vi "create_file_name (SubVI).vi"(0 "Use electrode config?":bool, 1 "Step Picomotors?":bool, 4 "picomotor index":i32, 6 "file_idx":i32, 8 "num files":i32, 9 "base name":string, 10 "Path":path, 11 "process_list":T2) -> (2 "filename_cluster":T1)   [LabVIEW 2018]
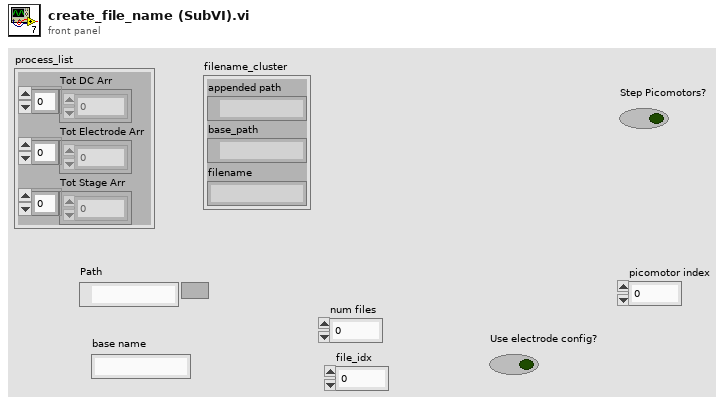
[diagram p1: front panel]
types:
  T1 = cluster{"appended path":path, "base_path":path, "filename":string}
  T2 = cluster{"Tot DC Arr":dbl[], "Tot Electrode Arr":dbl[], "Tot Stage Arr":dbl[]}
  T3 = cluster{"appended path":path, "path out":path, string}
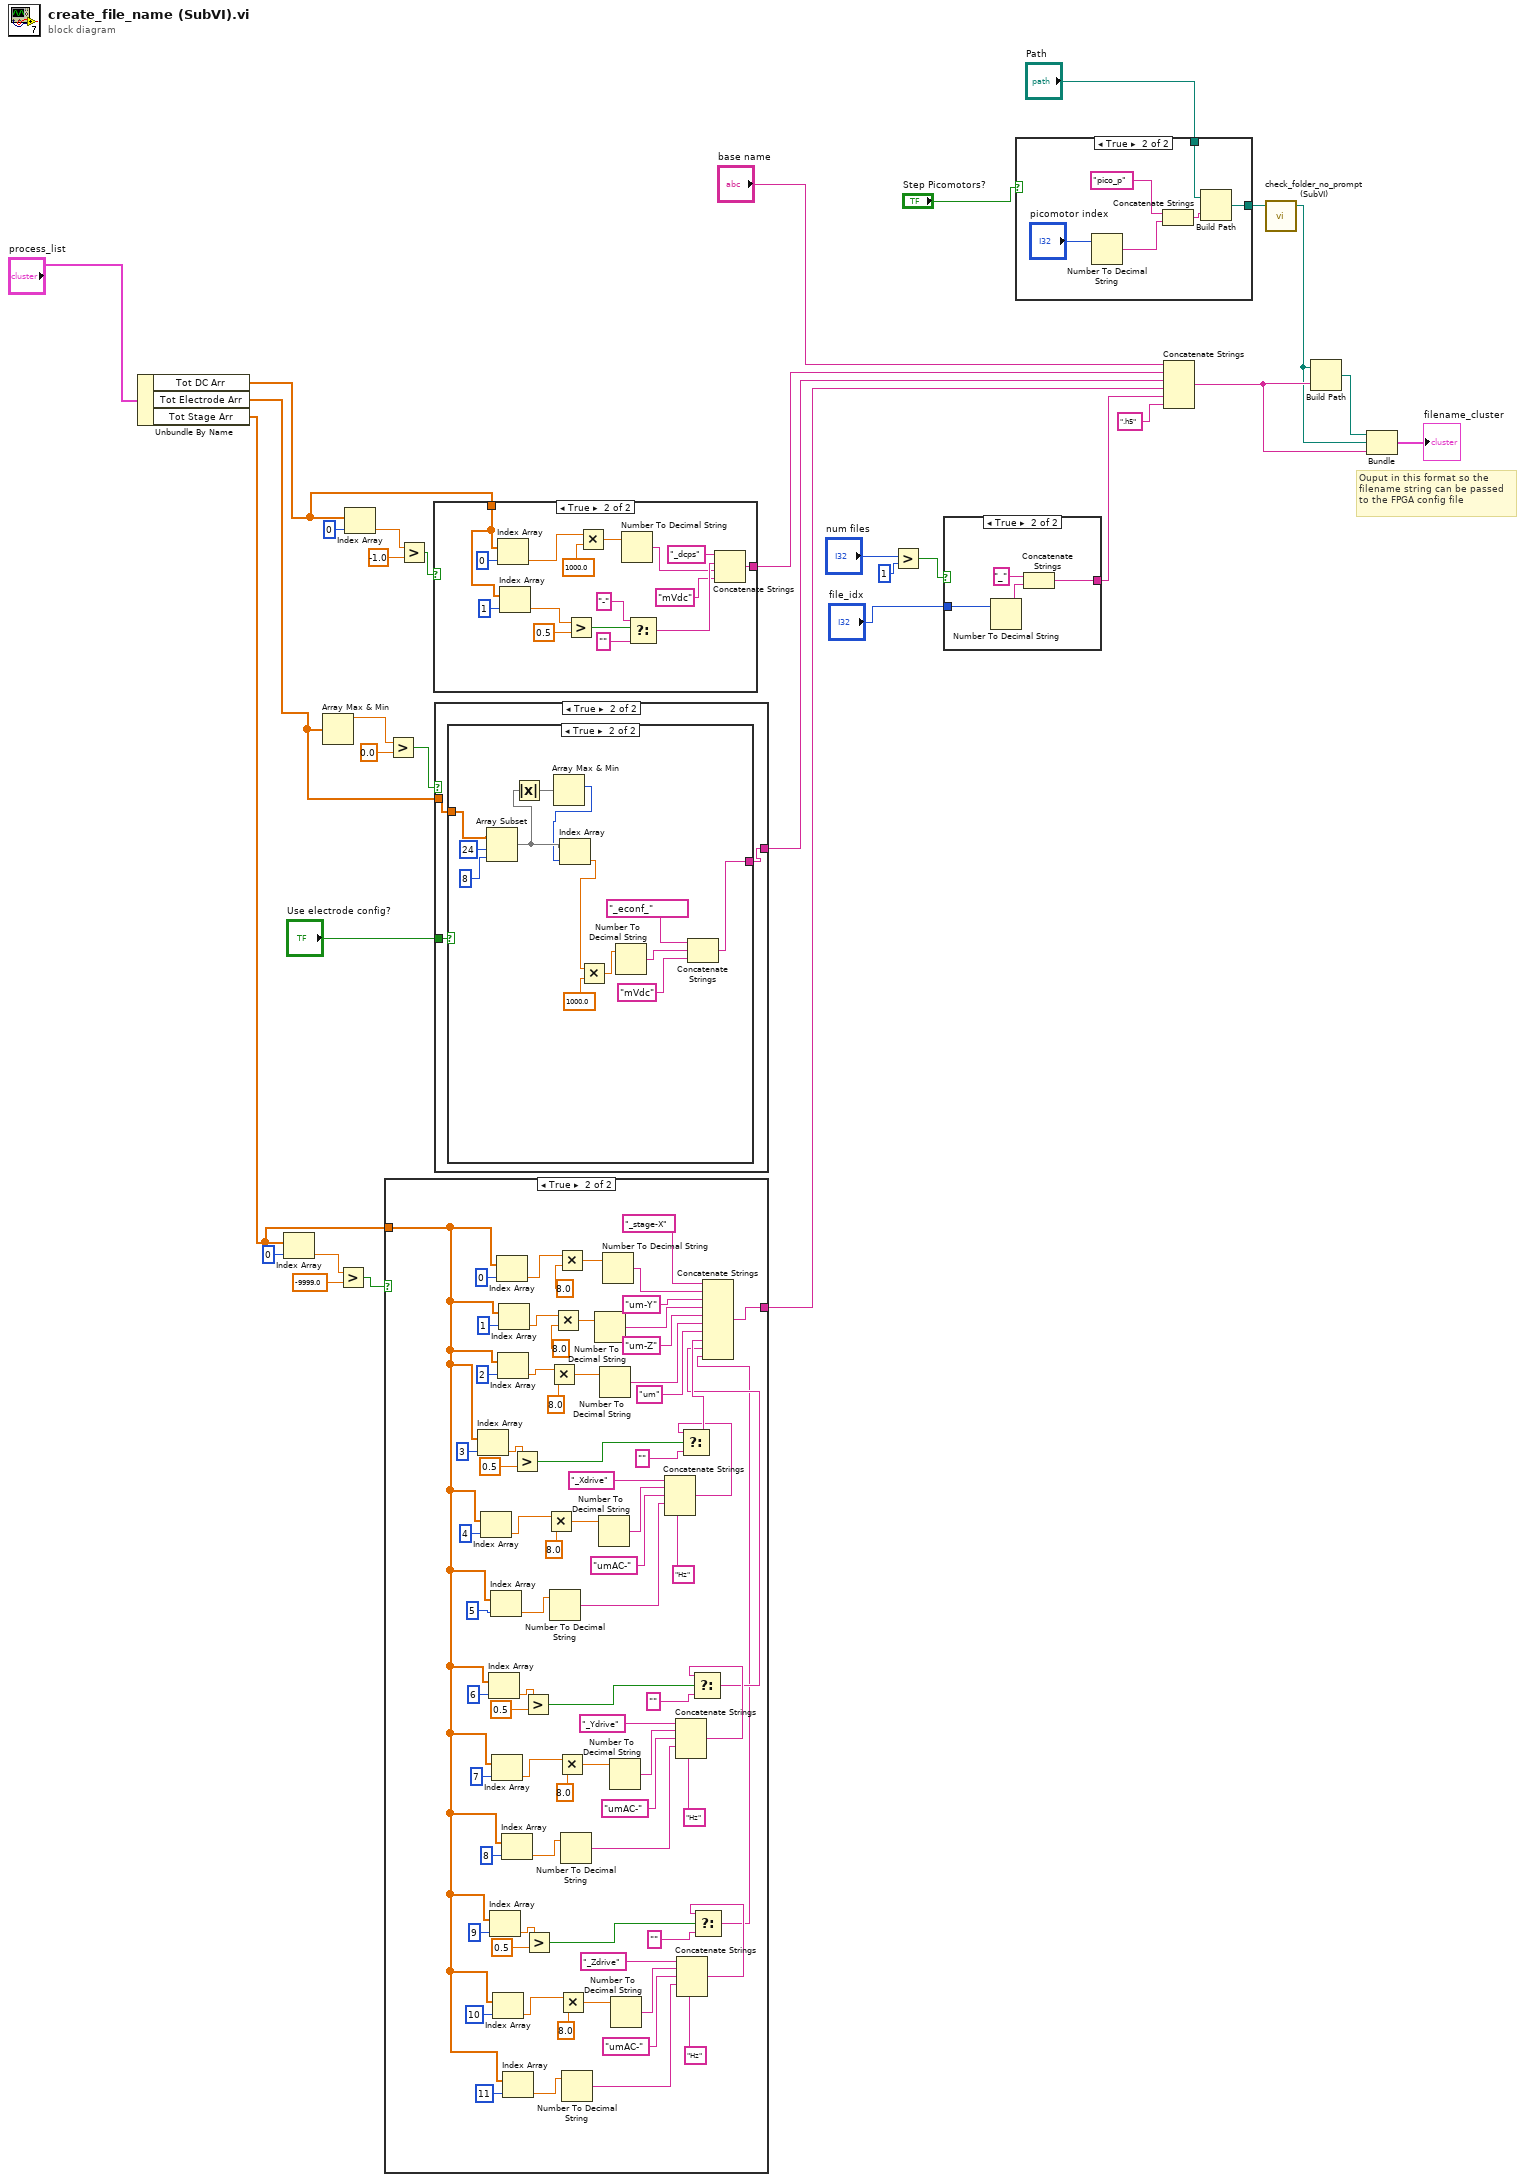
[diagram p0: block diagram]
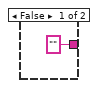
[diagram p3: hidden frame]
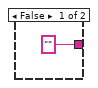
[diagram p4: hidden frame]
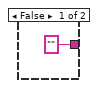
[diagram p5: hidden frame]
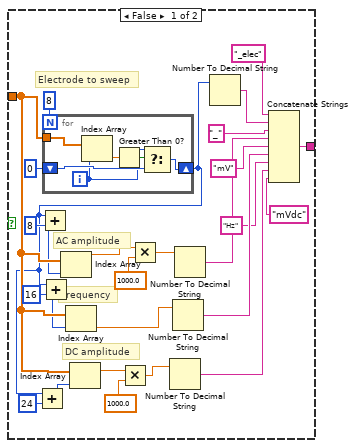
[diagram p6: hidden frame]
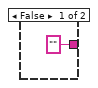
[diagram p7: hidden frame]
diagram:
  # "Ouput in this format so the\nfilename string can be passed\nto the FPGA config file"
  n1 = Unbundle By Name("process_list") -> ("Tot DC Arr"=w28:dbl[], "Tot Electrode Arr"=w11:dbl[], "Tot Stage Arr"=w21:dbl[])
  n2 = Index Array(array=w21, index=0) -> (element=w23:dbl)
  n3 = Array Max & Min(array=w11) -> (max value=w10:dbl)  [unwired: 3 out]
  n4 = Greater?(x=w23, y=-9999.0) -> (0:w22:bool)
  n5 = Index Array(array=w28, index=0) -> (element=w30:dbl)
  n6 = case shown="True" w22 {
    tunnel: w21 -> [_ w37]
    tunnel: ["" w90] -> w18
    frame False {
    }
    frame True {
      n7 = Index Array(array=w37, index=3) -> (element=w88:dbl)
      n8 = Index Array(array=w37, index=4) -> (element=w82:dbl)
      n9 = Index Array(array=w37, index=6) -> (element=w70:dbl)
      n10 = Index Array(array=w37, index=9) -> (element=w53:dbl)
      n11 = Index Array(array=w37, index=5) -> (element=w76:dbl)
      n12 = Index Array(array=w37, index=7) -> (element=w65:dbl)
      n13 = Index Array(array=w37, index=10) -> (element=w48:dbl)
      n14 = Index Array(array=w37, index=0) -> (element=w105:dbl)
      n15 = Index Array(array=w37, index=2) -> (element=w102:dbl)
      n16 = Index Array(array=w37, index=1) -> (element=w101:dbl)
      n17 = Index Array(array=w37, index=8) -> (element=w59:dbl)
      n18 = Index Array(array=w37, index=11) -> (element=w42:dbl)
      n19 = Greater?(x=w88, y=0.5) -> (0:w86:bool)
      n20 = Greater?(x=w70, y=0.5) -> (0:w68:bool)
      n21 = Greater?(x=w53, y=0.5) -> (0:w51:bool)
      n22 = Multiply(x=w82, y=8.0) -> (x*y=w80:dbl)
      n23 = Multiply(x=w102, y=8.0) -> (x*y=w98:dbl)
      n24 = Number To Decimal String(number=w76) -> (decimal integer string=w75:string)  [unwired: 1 in]
      n25 = Multiply(x=w101, y=8.0) -> (x*y=w99:dbl)
      n26 = Multiply(x=w105, y=8.0) -> (x*y=w100:dbl)
      n27 = Multiply(x=w65, y=8.0) -> (x*y=w63:dbl)
      n28 = Multiply(x=w48, y=8.0) -> (x*y=w46:dbl)
      n29 = Number To Decimal String(number=w59) -> (decimal integer string=w58:string)  [unwired: 1 in]
      n30 = Number To Decimal String(number=w42) -> (decimal integer string=w41:string)  [unwired: 1 in]
      n31 = Number To Decimal String(number=w99) -> (decimal integer string=w94:string)  [unwired: 1 in]
      n32 = Number To Decimal String(number=w80) -> (decimal integer string=w79:string)  [unwired: 1 in]
      n33 = Number To Decimal String(number=w98) -> (decimal integer string=w92:string)  [unwired: 1 in]
      n34 = Number To Decimal String(number=w100) -> (decimal integer string=w96:string)  [unwired: 1 in]
      n35 = Number To Decimal String(number=w63) -> (decimal integer string=w62:string)  [unwired: 1 in]
      n36 = Number To Decimal String(number=w46) -> (decimal integer string=w45:string)  [unwired: 1 in]
      n37 = Concatenate Strings("_Xdrive", w79, "umAC-" ("string"), w75, "Hz" ("string")) -> (w73:string)
      n38 = Concatenate Strings("_Ydrive", w62, "umAC-" ("string"), w58, "Hz" ("string")) -> (w56:string)
      n39 = Concatenate Strings("_Zdrive", w45, "umAC-" ("string"), w41, "Hz" ("string")) -> (w39:string)
      n40 = Select(t=w73, s=w86, f="" ("string")) -> (s? t:f=w84:string)
      n41 = Select(t=w56, s=w68, f="" ("string")) -> (s? t:f=w36:string)
      n42 = Select(t=w39, s=w51, f="" ("string")) -> (s? t:f=w35:string)
      n43 = Concatenate Strings("_stage-X", w96, "um-Y" ("string"), w94, "um-Z" ("string"), w92, "um" ("string"), w84, w36, w35) -> (w90:string)
    }
  }
  n44 = Greater?(x=w10, y=0.0) -> (0:w26:bool)
  n45 = Greater?(x=w30, y=-1.0) -> (0:w29:bool)
  n46 = case shown="True" w29 {
    tunnel: w28 -> [_ w124]
    tunnel: ["" w111] -> w20
    frame False {
    }
    frame True {
      n47 = Index Array(array=w124, index=0) -> (element=w122:dbl)
      n48 = Index Array(array=w124, index=1) -> (element=w118:dbl)
      n49 = Greater?(x=w118, y=0.5) -> (0:w117:bool)
      n50 = Multiply(x=w122, y=1000.0) -> (x*y=w121:dbl)
      n51 = Number To Decimal String(number=w121) -> (decimal integer string=w113:string)  [unwired: 1 in]
      n52 = Select(t="-" ("string"), s=w117, f="" ("string")) -> (s? t:f=w114:string)
      n53 = Concatenate Strings("_dcps" ("string"), w114, w113, "mVdc" ("string")) -> (w111:string)
    }
  }
  n54 = case shown="True" w26 {
    tunnel: w11 -> [_ w130]
    tunnel: ["" w129] -> w19
    tunnel: "Use electrode config?" -> [_ w128]
    frame False {
    }
    frame True {
      n55 = case shown="True" w128 {
        tunnel: w130 -> [w157 w174]
        tunnel: [w140 w175] -> w129
        frame False {
          # "DC amplitude"
          # "Frequency"
          # "AC amplitude"
          # "Electrode to sweep"
          n56 = for {
            N: 8 -> [_]
            tunnel: w157 -> [w163]
            shift-right: [w159] -> w132
            shift-left: 0 -> [w160]
            i -> [w158]
            n57 = Index Array(array=w163, index=w158) -> (element=w162:dbl)
            n58 = Greater Than 0?(x=w162) -> (x > 0?=w161:bool)
            n59 = Select(t=w158, s=w161, f=w160) -> (s? t:f=w159:i32)
          }
          n60 = Add(x=w132, y=24) -> (x+y=w133:i32)
          n61 = Add(x=w132, y=8) -> (x+y=w137:i32)
          n62 = Add(x=w132, y=16) -> (x+y=w135:i32)
          n63 = Index Array(array=w157, index=w137) -> (element=w151:dbl)
          n64 = Index Array(array=w157, index=w135) -> (element=w149:dbl)
          n65 = Index Array(array=w157, index=w133) -> (element=w148:dbl)
          n66 = Multiply(x=w148, y=1000.0) -> (x*y=w147:dbl)
          n67 = Multiply(x=w151, y=1000.0) -> (x*y=w150:dbl)
          n68 = Number To Decimal String(number=w147) -> (decimal integer string=w142:string)  [unwired: 1 in]
          n69 = Number To Decimal String(number=w149) -> (decimal integer string=w144:string)  [unwired: 1 in]
          n70 = Number To Decimal String(number=w150) -> (decimal integer string=w146:string)  [unwired: 1 in]
          n71 = Number To Decimal String(number=w132) -> (decimal integer string=w155:string)  [unwired: 1 in]
          n72 = Concatenate Strings("_elec" ("string"), w155, "_" ("string"), w146, "mV" ("string"), w144, "Hz" ("string"), w142, "mVdc" ("string")) -> (w140:string)
        }
        frame True {
          n73 = Array Subset(array=w174, index=24, length=8) -> (w166:dbl[])
          n74 = Absolute Value(x=w166) -> (abs(x)=w167:dbl[])
          n75 = Array Max & Min(array=w167) -> (max index (indices)=w164:i32)  [unwired: 3 out]
          n76 = Index Array(array=w166, index=w164) -> (element=w165:dbl)
          n77 = Multiply(x=w165, y=1000.0) -> (x*y=w170:dbl)
          n78 = Number To Decimal String(number=w170) -> (decimal integer string=w169:string)  [unwired: 1 in]
          n79 = Concatenate Strings("_econf_", w169, "mVdc" ("string")) -> (w175:string)
        }
      }
    }
  }
  n80 = Greater?(x="num files", y=1) -> (0:w15:bool)
  n81 = case shown="True" w15 {
    tunnel: "file_idx" -> [_ w180]
    tunnel: ["" w178] -> w13
    frame False {
    }
    frame True {
      n82 = Number To Decimal String(number=w180) -> (decimal integer string=w179:string)  [unwired: 1 in]
      n83 = Concatenate Strings("_" ("string"), w179) -> (w178:string)
    }
  }
  n84 = case shown="True" "Step Picomotors?" {
    tunnel: "Path" -> [w182 w185]
    tunnel: [w182 w184] -> w6
    frame False {
    }
    frame True {
      n85 = Number To Decimal String(number="picomotor index") -> (decimal integer string=w188:string)  [unwired: 1 in]
      n86 = Concatenate Strings("pico_p" ("string"), w188) -> (w186:string)
      n87 = Build Path(base path=w185, name or relative path=w186) -> (appended path=w184:path)
    }
  }
  n88 = Concatenate Strings("base name", w20, w19, w18, w13, ".h5" ("string")) -> (w4:string)
  n89 = call "check_folder_no_prompt (SubVI).vi"("path in"=w6) -> ("path out"=w3:path)  [unwired: 10 in]
  n90 = Build Path(base path=w3, name or relative path=w4) -> (appended path=w5:path)
  n91 = Bundle("appended path"=w5, "path out"=w3, w4) -> (→"filename_cluster":T3)  [unwired: 1 in]
